vi "PTScanner.edit object.vi"(0 "i ref in":refnum<vi>, 2 "Parameters":T1, 4 "index":i32, 5 "error in (no error)":errorcluster) -> (14 "i ref out":refnum<vi>, 19 "error out":errorcluster)   [LabVIEW 2014, in "PTScanner.lvlib"]
uses:
  PTScanner.lvlib
  PTScanner.obj parameters.ctl
  CSlibraries-extern/DimLVEvent/LVDimInterface/LVDimInterface.lvlib
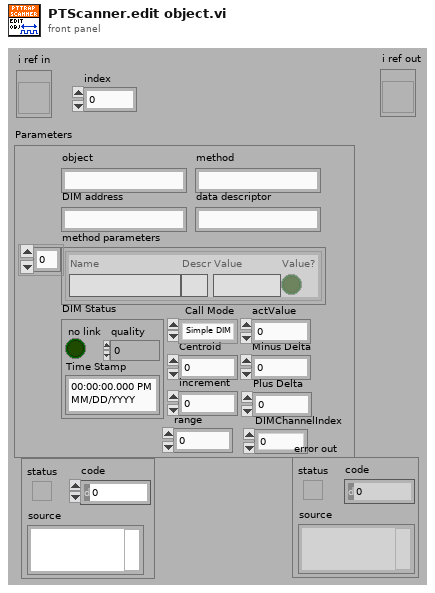
[diagram p1: front panel]
types:
  T1 = typedef "PTScanner.lvlib/PTScanner.obj parameters.ctl" = cluster{"object":string, "DIM address":string, "method":string, "data descriptor":string, "method parameters":cluster{"Name":string, "Descr":string, "Value":string, "Value?":bool}[], "Call Mode":enum16{"Simple DIM", "Synchronous"}, "actValue":dbl, "Centroid":dbl, "Minus Delta":dbl, "Plus Delta":dbl, "increment":dbl, "DIM Status":cluster{"no link":bool, "quality":i32, "Time Stamp":timestamp}, "range":dbl, "DIMChannelIndex":i32}
  T2 = typedef "PTScanner.lvlib/PTScanner.i attribute.ctl" = cluster{"Object cmds":T1[], "Steps":cluster{"Finished":bool, "cmd setup":T3[]}[], "curStep":i32, "DIM IDs":cluster{"AllFinished":i32, "Finished":i32, "curStep":i32, "nofSteps":i32, "NomValues":i32[], "1D-Min":i32, "1D-Max":i32, "Dimensions":i32, "MaxDimensions":i32, "ScanedDeviceNames":i32[]}, "All Finished":bool, "DIMs in use":string[], "Running":bool, "Scan Delay":u32, "loop":bool, "Paused":bool, "Formed":bool}
  T3 = typedef "PTScanner.lvlib/PTScanner.step obj parameters.ctl" = cluster{"obj index":i32, "nomValue":dbl, "fulfilled":bool}
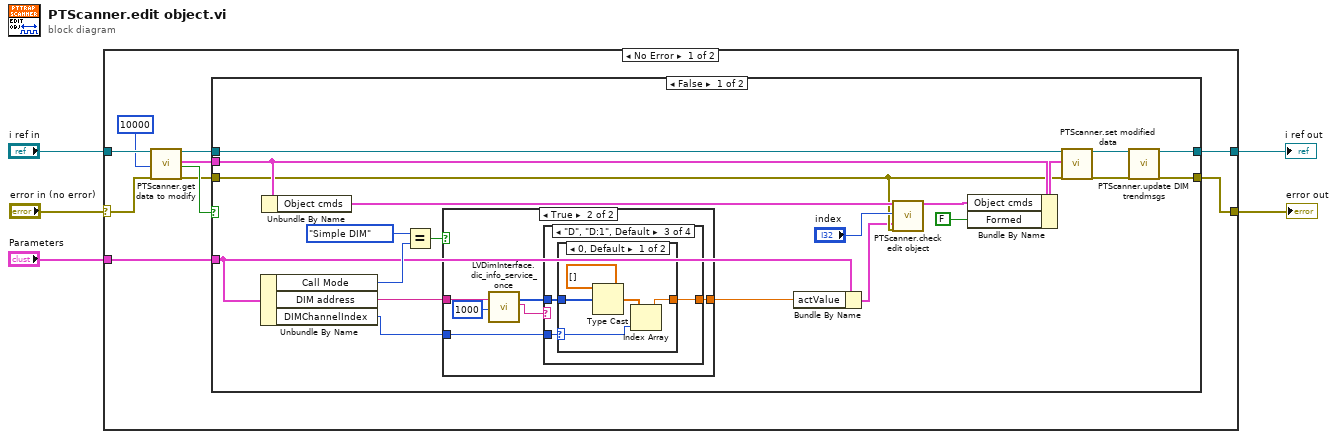
[diagram p0: block diagram]
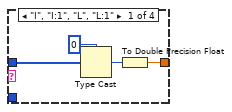
[diagram p3: hidden frame]
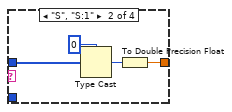
[diagram p4: hidden frame]
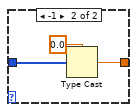
[diagram p5: hidden frame]
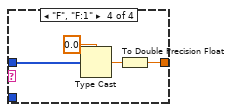
[diagram p6: hidden frame]
diagram:
  n1 = case shown="No Error" "error in (no error)" {
    selector: "error in (no error)" -> [w10 w67]
    tunnel: "i ref in" -> [w11 w68]
    tunnel: [w9 w68] -> w3
    tunnel: [w7 w67] -> w2
    tunnel: "Parameters" -> [w6 _]
    frame No Error {
      n2 = call "PTScanner.get data to modify.vi"("i ref in"=w11, "ms timeout (10000)"=10000, "error in (no error)"=w10) -> ("i ref out"=w14:refnum<vi>, "i attribute"=w12:T2, "timed out"=w15:bool, "error out"=w13:errorcluster)  [unwired: 13 in]
      n3 = case shown="False" w15 {
        tunnel: w14 -> [w35 w65]
        tunnel: w13 -> [w22 w66]
        tunnel: w12 -> [w34 _]
        tunnel: [w27 w66] -> w7
        tunnel: [w28 w65] -> w9
        tunnel: w6 -> [w19 _]
        frame False {
          n4 = Unbundle By Name(w19) -> ("Call Mode"=w21:enum16{"Simple DIM", "Synchronous"}, "DIM address"=w20:string, "DIMChannelIndex"=w16:i32)
          n5 = Unbundle By Name(w34) -> ("Object cmds"=w25:T1[])
          n6 = Equal?(x=enum16{"Simple DIM", "Synchronous"}."Simple DIM" ("Call Mode"), y=w21) -> (x = y?=w30:bool)
          n7 = case shown="True" w30 {
            tunnel: [_ w38] -> w18
            tunnel: w20 -> [_ w37]
            tunnel: w16 -> [_ w36]
            frame False {
            }
            frame True {
              n8 = call "LVDimInterface.dic_info_service_once.vi"("serviceName"=w37, "timeout [ms]"=u32 1000) -> ("data"=w39:i8[], "typeDescriptor"=w40:string)  [unwired: 14 in, 2 out]
              n9 = case shown="\"D\", \"D:1\", Default" w40 {
                tunnel: w39 -> [w44 w48 w52 w63]
                tunnel: [w42 w46 w51 w61] -> w38
                tunnel: w36 -> [_ _ w50 _]
                frame "I", "I:1", "L", "L:1" {
                  n10 = Type Cast(type=0, x=w44) -> (*(type *) &x=w43:i32)
                  n11 = To Double Precision Float(number=w43) -> (double precision float=w42:dbl)
                }
                frame "S", "S:1" {
                  n12 = Type Cast(type=i16 0, x=w48) -> (*(type *) &x=w47:i16)
                  n13 = To Double Precision Float(number=w47) -> (double precision float=w46:dbl)
                }
                frame "D", "D:1", Default {
                  n14 = case shown="0, Default" w50 {
                    selector: w50 -> [w53 _]
                    tunnel: w52 -> [w56 w59]
                    tunnel: [w54 w58] -> w51
                    frame 0, Default {
                      n15 = Type Cast(type=dbl[] [], x=w56) -> (*(type *) &x=w55:dbl[])
                      n16 = Index Array(array=w55, index=w53) -> (element=w54:dbl)
                    }
                    frame -1 {
                      n17 = Type Cast(type=0.0, x=w59) -> (*(type *) &x=w58:dbl)
                    }
                  }
                }
                frame "F", "F:1" {
                  n18 = Type Cast(type=sgl 0.0, x=w63) -> (*(type *) &x=w62:sgl)
                  n19 = To Double Precision Float(number=w62) -> (double precision float=w61:dbl)
                }
              }
            }
          }
          n20 = Bundle By Name(cluster=w19, "actValue"=w18) -> (w17:T1)
          n21 = call "PTScanner.check edit object.vi"("Object cmds"=w25, "index"="index", "new obj command"=w17, "error in (no error)"=w22) -> ("Object cmds out"=w24:T1[])  [unwired: 14 in, 1 out]
          n22 = Bundle By Name(cluster=w34, "Object cmds"=w24, "Formed"=FALSE) -> (w33:T2)
          n23 = call "PTScanner.set modified data.vi"("i ref in"=w35, "CLASS.i attribute"=w33, "error in (no error)"=w22) -> ("i ref out"=w29:refnum<vi>, "error out"=w26:errorcluster)  [unwired: 15 in]
          n24 = call "PTScanner.update DIM trendmsgs.vi"("i ref in"=w29, "error in"=w26) -> ("i ref out"=w28:refnum<vi>, "error out"=w27:errorcluster)  [unwired: 16 in]
        }
        frame True {
        }
      }
    }
    frame Error {
    }
  }
  "i ref out" <- w3
  "error out" <- w2
